vi "subdev spec pairs equal.vi"(8 "error in (no error)":errorcluster, 9 "result_out":i32, 10 "second":cluster{"db_name":u64, "sd_name":u64}, 11 "first":cluster{"db_name":u64, "sd_name":u64}) -> (0 "error out":errorcluster, 1 "result_out out":i32, 3 "function return":u32(ring))   [LabVIEW 2023, in "uhd.lvlib"]
doc: "UHD_API uhd_error uhd_subdev_spec_pairs_equal(const uhd_subdev_spec_pair_t* first,\n const uhd_subdev_spec_pair_t* second,\n bool* result_out);"
uses:
  <userlib>/uhd/uhd.lvlib
  <userlib>/uhd/uhd.dll
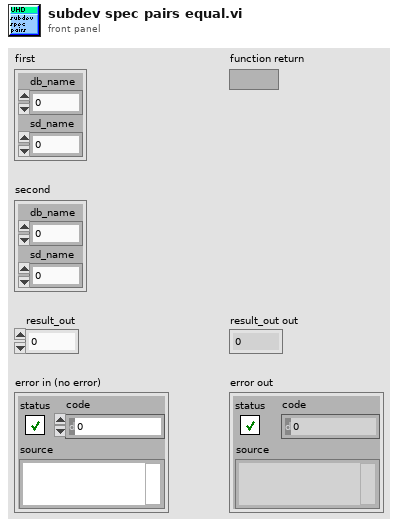
[diagram p1: front panel]
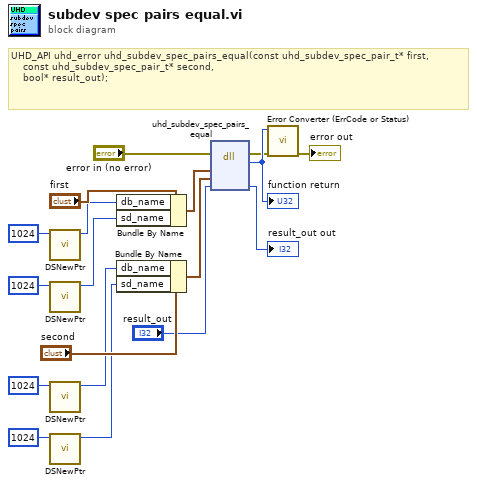
[diagram p0: block diagram]
diagram:
  # "UHD_API uhd_error uhd_subdev_spec_pairs_equal(const uhd_subdev_spec_pair_t* first,\n    const uhd_subdev_spec_pair_t* second,\n    bool* result_out);"
  n1 = call <vilib>:"DSNewPtr.vi"("Size"=u64 1024) -> ("Pointer"=w14:u64)  [unwired: 9 in, 1 out]
  n2 = call <vilib>:"DSNewPtr.vi"("Size"=u64 1024) -> ("Pointer"=w12:u64)  [unwired: 9 in, 1 out]
  n3 = call <vilib>:"DSNewPtr.vi"("Size"=u64 1024) -> ("Pointer"=w8:u64)  [unwired: 9 in, 1 out]
  n4 = call <vilib>:"DSNewPtr.vi"("Size"=u64 1024) -> ("Pointer"=w6:u64)  [unwired: 9 in, 1 out]
  n5 = Bundle By Name(cluster="first", "db_name"=w14, "sd_name"=w12) -> (w13:cluster{"db_name":u64, "sd_name":u64})
  n6 = Bundle By Name(cluster="second", "db_name"=w8, "sd_name"=w6) -> (w7:cluster{"db_name":u64, "sd_name":u64})
  n7 = dll-call lib="C:/Program Files/National Instruments/LabVIEW 2023/user.lib/uhd/uhd.*" fn="uhd_subdev_spec_pairs_equal"(error in="error in (no error)", "first"=w13, "second"=w7, "result_out"="result_out") -> (error out=w2:errorcluster, w18:u32, "result_out"=→"result_out out":i32)  [unwired: 4 in, 1 out]
  "function return" <- w18
  n8 = call <userlib>:"Error Converter (ErrCode or Status).vi"("error in (no error)"=w2, "error code"=w18) -> ("error out"=→"error out":errorcluster)  [unwired: 9 in]
